vi "ACCES device lookup.vi"(5 "ReInit?":bool, 7 "file path (use dialog)":path, 8 "error in (no error)":errorcluster, 10 "Device Code":u32) -> (0 "error out":errorcluster, 2 "error message (\"\")":string)   [LabVIEW 2012]
doc: "Loops up a board name by product ID"
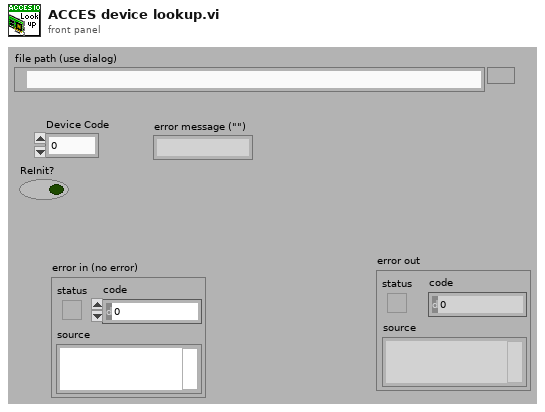
[diagram p1: front panel]
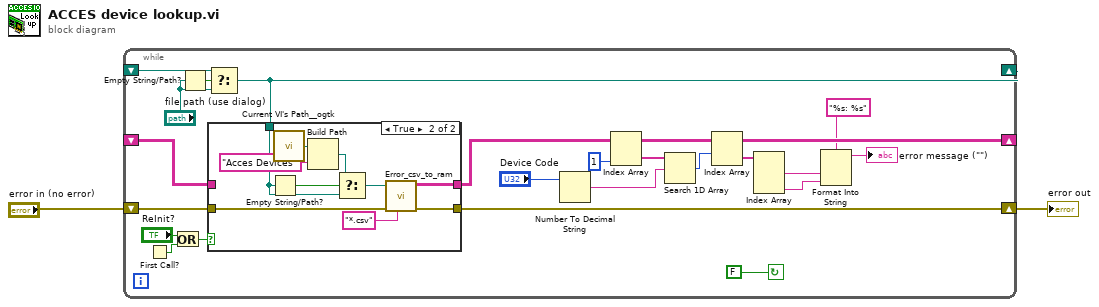
[diagram p0: block diagram]
diagram:
  n1 = while {
    shift-right: [w22] -> w1
    shift-left: "error in (no error)" -> [w23]
    shift-right: [w20] -> _
    shift-left: _ -> [w21]
    shift-right: [w9] -> _
    shift-left: _ -> [w14]
    stop <- FALSE continue-if-true
    n2 = First Call?() -> (First Call?: T/F=w16:bool)
    n3 = Or(x="ReInit?", y=w16) -> (x .or. y?=w17:bool)
    n4 = Empty String/Path?(string/path="file path (use dialog)") -> (empty?=w19:bool)
    n5 = Select(t=w21, s=w19, f="file path (use dialog)") -> (s? t:f=w20:path)
    n6 = case shown="True" w17 {
      tunnel: w23 -> [w26 w36]
      tunnel: [w26 w35] -> w22
      tunnel: w20 -> [_ w32]
      tunnel: [w25 w34] -> w9
      tunnel: w14 -> [w25 _]
      frame False {
      }
      frame True {
        n7 = Empty String/Path?(string/path=w32) -> (empty?=w33:bool)
        n8 = call "Current VI's Path__ogtk.vi"() -> ("Current VI's Path (+ Relative)"=w30:path)  [unwired: 1 in]
        n9 = Build Path(base path=w30, name or relative path="Acces Devices") -> (appended path=w29:path)
        n10 = Select(t=w29, s=w33, f=w32) -> (s? t:f=w31:path)
        n11 = call "Error_csv_to_ram.vi"("pattern"="*.csv", "error in (no error)"=w36, "file path (use dialog)"=w31) -> ("error out"=w35:errorcluster, "array"=w34:string[][])  [unwired: 7 in]
      }
    }
    n12 = Number To Decimal String(number="Device Code") -> (decimal integer string=w10:string)  [unwired: 1 in]
    n13 = Index Array(array=w9, index (col)=1 ("disabled index (col)")) -> (element=w13:string[])  [unwired: 1 in]
    n14 = Search 1D Array(1D array=w13, element=w10) -> (index of element=w8:i32)  [unwired: 1 in]
    n15 = Index Array(array=w9, index (row)=w8) -> (element=w7:string[])  [unwired: 1 in]
    n16 = Index Array(array=w7) -> (element #1=w6:string, element #3=w5:string)  [unwired: 3 in, 1 out]
    n17 = Format Into String(format string="%s: %s", w6, w5) -> (resulting string=→"error message (\"\")":string)  [unwired: 2 in, 1 out]
  }
  "error out" <- w1
